vi "Insert (array).vi"(8 "error in (no error)":errorcluster, 10 "Array of Pairs":T1[](array[typedef]), 11 "Parameter to Hardware Map in":refnum<class "Parameter to Hardware Map.lvclass">) -> (0 "error out":errorcluster, 3 "Parameter to Hardware Map out":refnum<class "Parameter to Hardware Map.lvclass">)   [LabVIEW 2020, in "RxnRover.lvlib" / "Parameter to Hardware Map.lvclass"]
doc: "Insert the given key-value pairs into the map."
uses:
  Parameter to Hardware Map.lvclass
  Pair.ctl
  Controller/Generic Plugin.lvclass
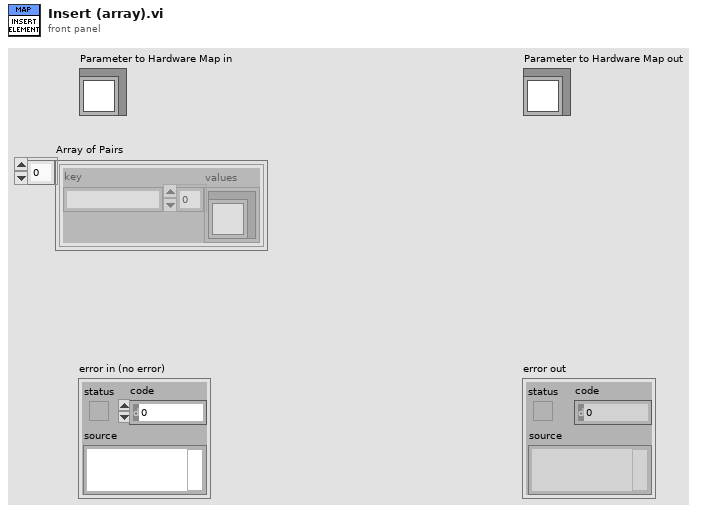
[diagram p1: front panel]
types:
  T1 = typedef "RxnRover.lvlib/Parameter to Hardware Map.lvclass/Pair.ctl" = cluster{"key":string, "values":refnum<class "Generic Plugin.lvclass">[]}
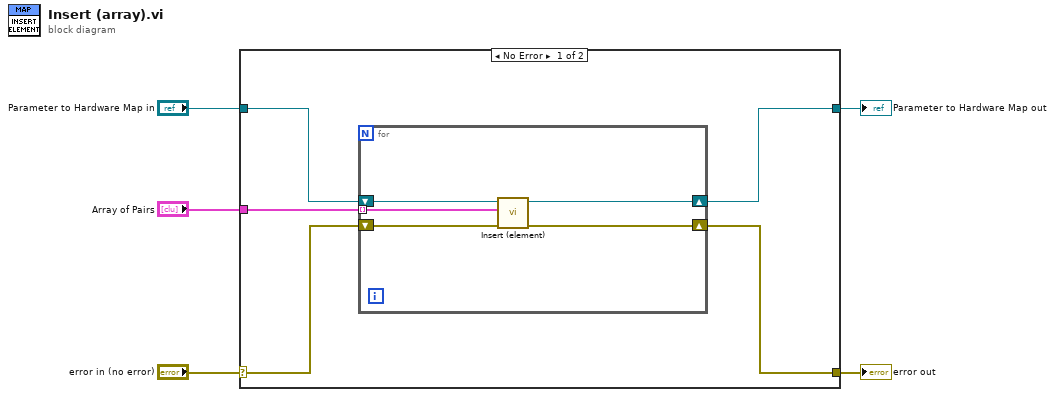
[diagram p0: block diagram]
diagram:
  n1 = case shown="No Error" "error in (no error)" {
    selector: "error in (no error)" -> [w9 w17]
    tunnel: [w7 w17] -> w4
    tunnel: [w6 w16] -> w2
    tunnel: "Parameter to Hardware Map in" -> [w10 w16]
    tunnel: "Array of Pairs" -> [w8 _]
    frame No Error {
      n2 = for {
        tunnel: w8 -> [w13] mode=indexing
        shift-right: [w11] -> w6
        shift-left: w10 -> [w12]
        shift-right: [w14] -> w7
        shift-left: w9 -> [w15]
        n3 = call "Insert (element).vi"("error in (no error)"=w15, "Key-Value Pair"=w13, "Parameter to Hardware Map in"=w12) -> ("error out"=w14:errorcluster, "Parameter to Hardware Map out"=w11:refnum<class "Parameter to Hardware Map.lvclass">)  [unwired: 7 in]
      }
    }
    frame Error {
    }
  }
  "error out" <- w4
  "Parameter to Hardware Map out" <- w2
